vi "CloseXL_Workbook.vi"(6 "Save? (F)":bool, 8 "error in (no error)":errorcluster, 11 "Refnum Cluster In":T1) -> (0 "error out":errorcluster, 3 "Refnum Cluster Out":T2)   [LabVIEW 2017, in "excel_configuration.lvlib"]
doc: "Closes the open Excel workbook and releases the workbook reference. Set Save? (F) to save the workbook before closing."
uses:
  excel_configuration.lvlib
  648d9216-624b-4798-a9d5-a0399acbd7d7.vi
  <vilib>/Utility/error.llb/Clear Errors.vi
panel:
  in  "path":path
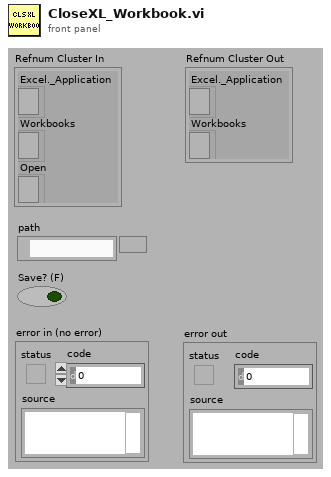
[diagram p1: front panel]
types:
  T1 = cluster{"Excel._Application":refnum<k7>, "Workbooks":refnum<k7>, "Open":refnum<k7>}
  T2 = cluster{"Excel._Application":refnum<k7>, "Workbooks":refnum<k7>}
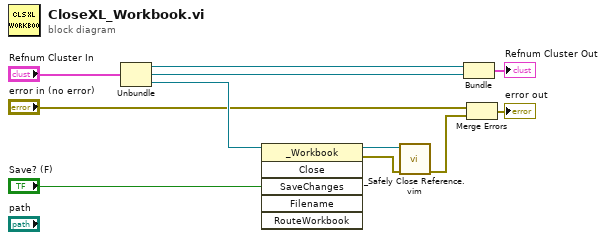
[diagram p0: block diagram]
diagram:
  n1 = Unbundle("Refnum Cluster In") -> ("Excel._Application"=w7:refnum<k7>, "Workbooks"=w6:refnum<k7>, "Open"=w5:refnum<k7>)
  n2 = invoke class="_Workbook" method="Close"(reference=w5, "SaveChanges"="Save? (F)") -> (reference out=w10:refnum<k7>, error out=w11:errorcluster)  [unwired: 4 in, 4 out]
  n3 = call "_Safely Close Reference.vim"("error in (no error)"=w11, "Automation Refnum in"=w10) -> ("error out"=w9:errorcluster)  [unwired: 9 in]
  n4 = Bundle("Excel._Application"=w7, "Workbooks"=w6) -> (→"Refnum Cluster Out":T2)  [unwired: 1 in]
  n5 = Merge Errors("error in (no error)", w9) -> (→"error out":errorcluster)
